vi "winchcontrol.vi"() -> ()   [LabVIEW 2009]
uses:
  Instance           1 20Saved   winchcontrol .vi
  Instance           2 20Saved   winchcontrol .vi
  Instance           4 20Saved   winchcontrol .vi
  Instance           3 20Saved   winchcontrol .vi
  Instance           5 20Saved   winchcontrol .vi
  Instance           6 20Saved   winchcontrol .vi
panel:
  out "Last update string":string
  in  "Port":i32=4050
  in  "Red Lion IP Address":string="192.168.1.160"
  in  "Beep\non wait?":bool=TRUE
  in  "Drive by \nCTD Data":bool
  out "isMaxPaySet":bool
  out "Old Max Payout":dbl
  in  "Maximum depth [m]":dbl=1000.0 min=0.0 max=2000.0 step=1.0 format="%#_4f"
  out "Time @ max":timestamp format="%<%H:%M:%S>T"
  out "Max payout":dbl format="%#_6f"
  out "Max depth":dbl format="%#_6f"
  in  "Go Up Now":bool
  in  "EMERGENCY\n      STOP":bool=TRUE caption="STOP!!!!!"
  in  "Final In Speed\n[turns/sec]":dbl=1.0 min=0.0 max=4.0 step=0.1 format="%_2f"
  in  "Slow depth\n[turns]":dbl=28.0 min=0.0 max=1500.0 step=1.0
  out "Final in Speed":dbl=3.0 min=0.0 max=4.0 step=0.1 format="%3_2g"
  out "Slow Depth":dbl=3.0 min=0.0 max=4.0 step=0.1
  out "Depth Derivative":dbl(graph)=-0.55843
  out "CTD Com Miss Count":dbl
  out "Winch Com Miss Count":dbl
  out "Sax Status":u8[](array[numeric])
  out "Pressure":dbl(graph)=-0.55843
  out "i value":i32
  out "concatenated string":string="$OPGST,1,2,1243"
  out "CTD data":string
  out "Depth":dbl(slide) min=0.0 max=1200.0 scale=2000.0..0.0 scale format="%#_4f"
  out "*(type *) &x":i32
  out "timestamp":u32=919485956
  out "Temperature":dbl(graph)=24.730053
  out "Parameter String":string="$OPGWPM,10,10,+0000,+0030,03,03,15000,15000,30000,30000,60000,60000,;"
  out "Status String":string="$OPGWST,1,0,2710.5,2710.5,0000, 00.00,-02,0000,ElmoStatusxxxxxx,;"
  out "Sax Status Code":dbl format="%#_8f"
  out "Motor Current":dbl=-2.0
  out "Motor Payout":dbl=2710.5
  out "Sheave Payout":dbl
  out "ATM90 Payout":dbl=2710.5
  in  "CTD Data  IP Address":string="192.168.1.158"
  in  "Port":i32=2342
  out "bytes written":i32
  out "RL Status Received":bool=TRUE
  out "Acc Out":dbl=15000.0
  out "Acc In":dbl=15000.0
  out "Winch Action Status":T1(ring)
  out "Winch Control Mode":T2(ring)=enum."MANUAL JOY"
  out "Decel Stop In":dbl=60000.0
  out "Decel Stop Out":dbl=60000.0
  out "Decel In":dbl=30000.0
  out "Decel Out":dbl=30000.0
  out "Wire In Speed":dbl=3.0
  out "Wire Out Speed":dbl=3.0
  out "Min Payout":dbl
  out "Max Payout":dbl=30.0
  out "I Limit Out":dbl=10.0
  out "I Limit In":dbl=10.0
  in  "Drop time [min.]":dbl=23.0 min=0.0 step=0.1 format="%.1f"
  out "output":string
  in  "Stop Now":bool
  in  "Wire In Speed\n[turns/sec]":dbl=2.8 min=0.0 max=5.0 step=0.1 format="%3_2f"
  in  "Decel in":dbl=30000.0
  in  "Decel out":dbl=30000.0
  in  "Stop decel in":dbl=60000.0
  in  "Stop decel out":dbl=60000.0
  in  "Accel  in":dbl=15000.0
  in  "Accel out":dbl=15000.0
  in  "Current limit out\n[Amps]":dbl=10.0 min=0.0 max=20.0 step=0.1 format="%_3f"
  in  "Current limit in\n[Amps]":dbl=16.0 min=0.0 max=18.0 format="%_3f"
  out "input 2":string="$OPGWPM,10,10,+0000,+0030,03,03,15000,15000,30000,30000,60000,60000,;"
  out "Depth History":cluster{"Depth":dbl, "Value":dbl}(graph)={"Depth"=0.0, "Value"=2710.5}
  out "Payout":dbl(slide)=97.75967413441958 min=0.0 max=1200.0 step=200.0 scale=2000.0..0.0 scale format="%#1_3f"
  out "Velocity Now":dbl(knob) min=-5.0 max=5.0 step=1.0 scale=-5.0..5.0 scale format="%#_1f"
  in  "Maximum payout [turns]":dbl=1500.0 min=0.0 max=1640.0 step=1.0 format="%#_4f"
  in  "Minimum payout [turns]":dbl=30.0 min=0.0 max=2000.0 step=1.0
  in  "Winch Auto Run":bool
  out "Enabled":bool
  in  "Wire Out Speed\n[turns/sec]":dbl=4.0 min=0.0 max=5.0 step=0.1 format="%_2f"
  out "Target\nDepth":dbl
  out "Conductivity":dbl(graph)=1e-06
  # "OPG  FAST  CTD"
  # "Winch Variable Status"
  # "Winch Variable Controls"
  # "FCTD DATA COMMUNICATION SETUP"
  # "RED LION CONTROL PANEL COM."
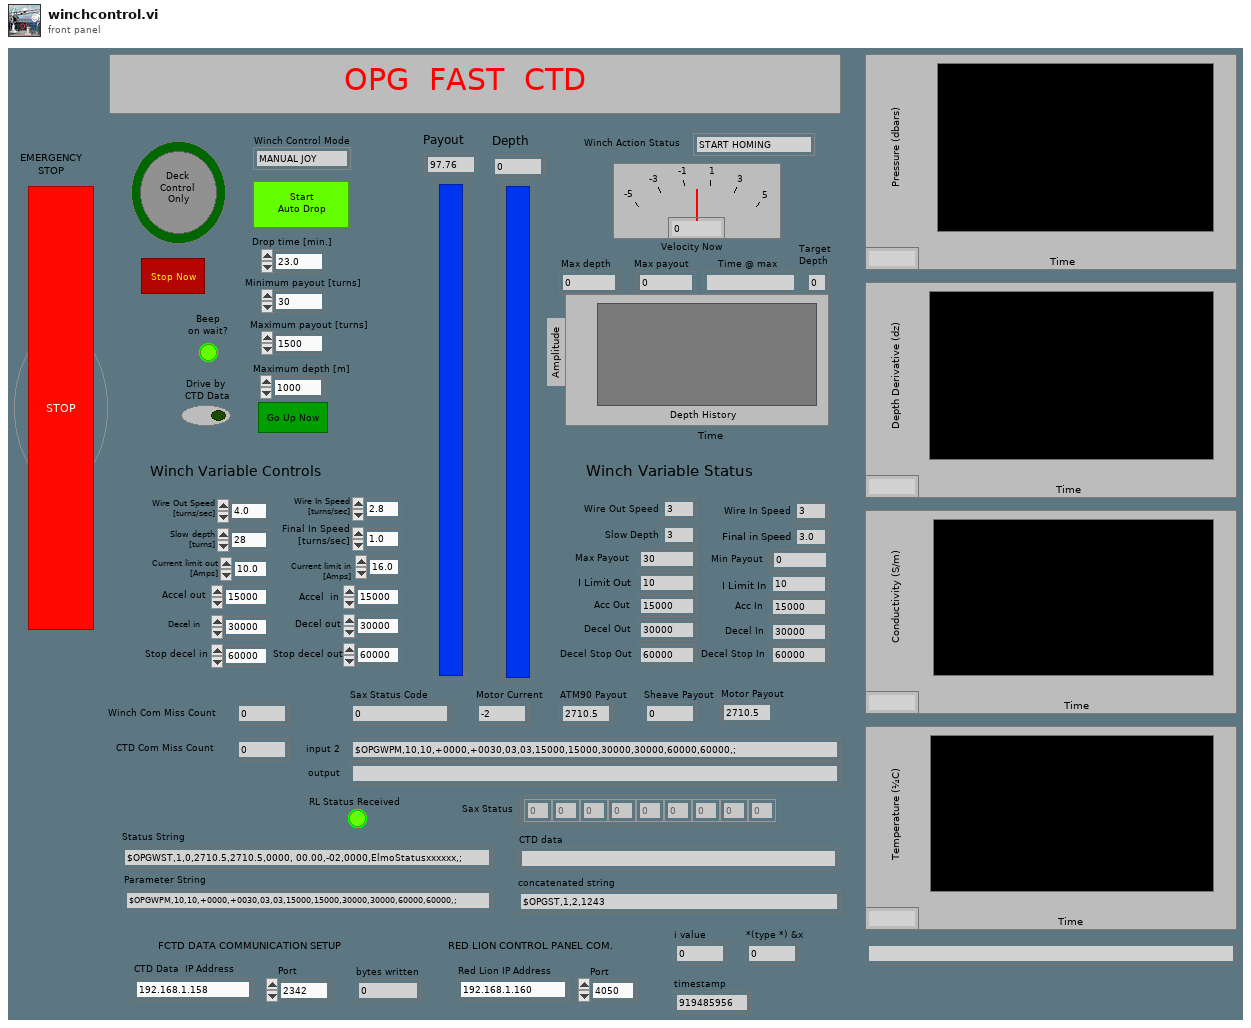
[diagram p1: front panel]
types:
  T1 = enum16{"START HOMING", "HOMING", "WAIT FOR TRIGGER", "START DROP", "GOING DOWN ?", "GOING UP"}
  T2 = enum16{"STOPPED", "MANUAL JOY", "MANUAL POT", "AUTO", "SEMIAUTO"}
  T3 = cluster{"Array[0]":dbl, "Array[1]":dbl, "Array[2]":dbl, "Array[3]":dbl, "Array[4]":dbl, "Array[5]":dbl, "Array[6]":dbl, "Array[7]":dbl, "Array[8]":dbl}
  T4 = cluster{"Array[0]":dbl, "Array[1]":dbl, "Array[2]":dbl, "Array[3]":dbl, "Array[4]":dbl, "Array[5]":dbl, "Array[6]":dbl, "Array[7]":dbl, "Array[8]":dbl, "Array[9]":dbl, "Array[10]":dbl, "Array[11]":dbl, "Array[12]":dbl, "Array[13]":dbl}
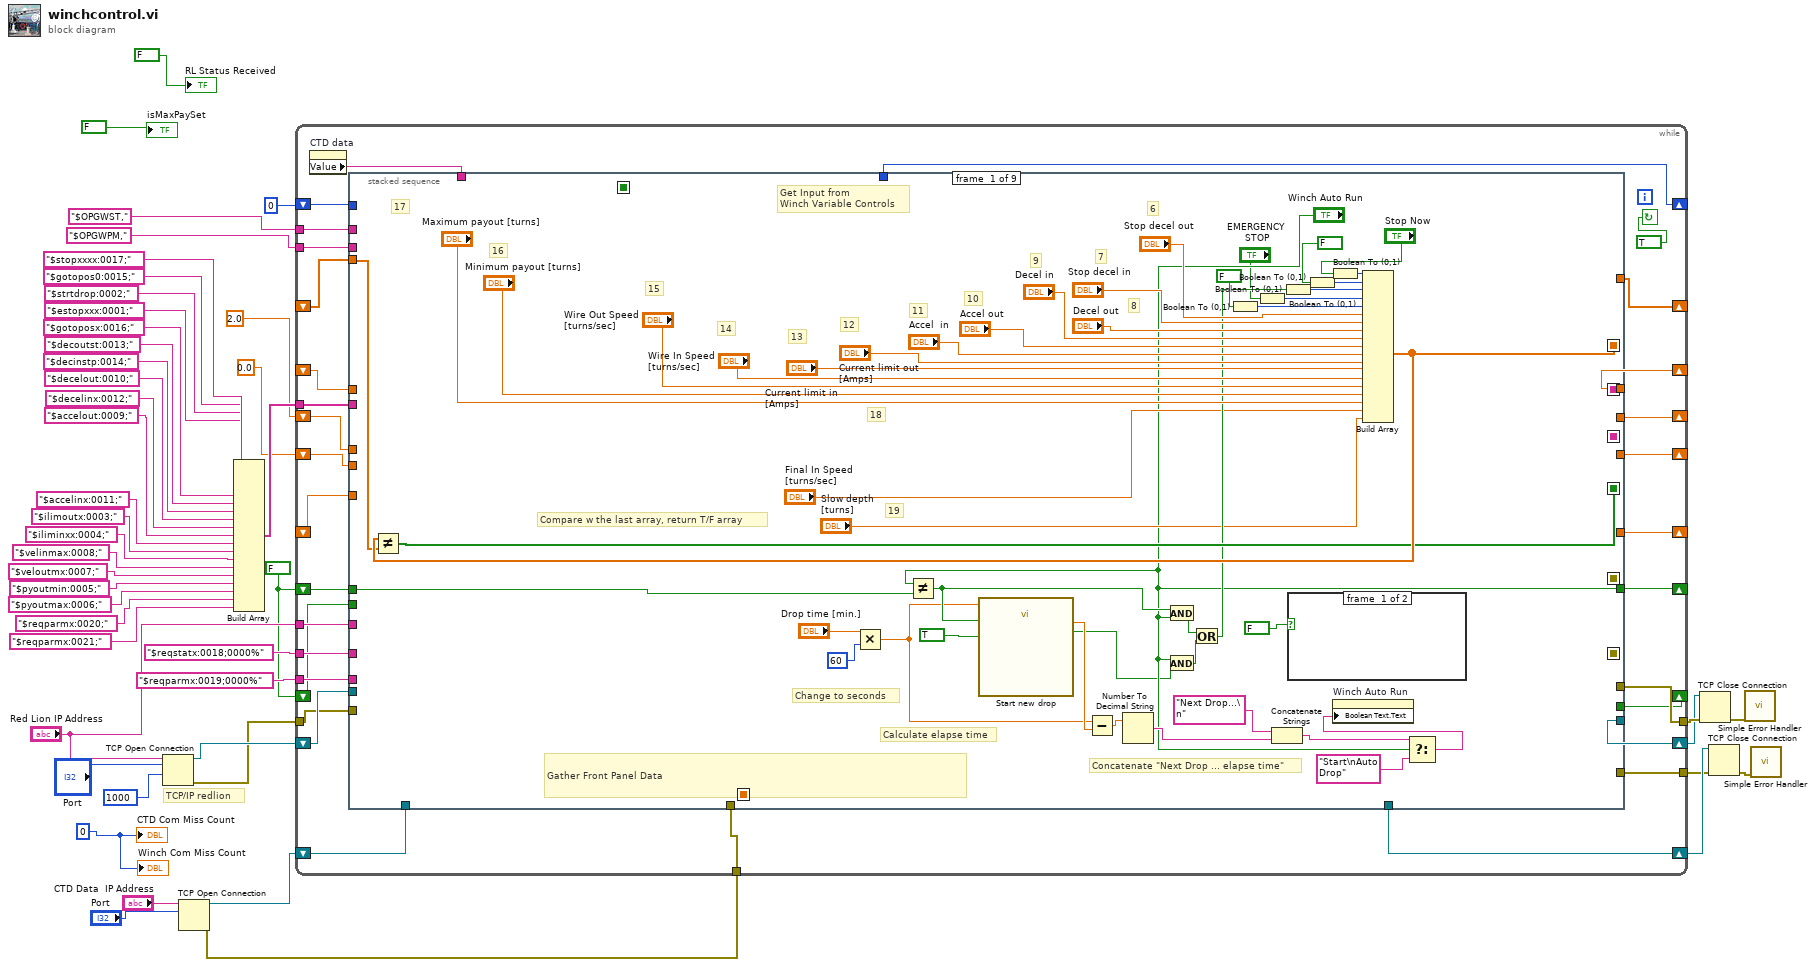
[diagram p0: block diagram]
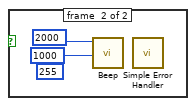
[diagram p2: hidden frame]
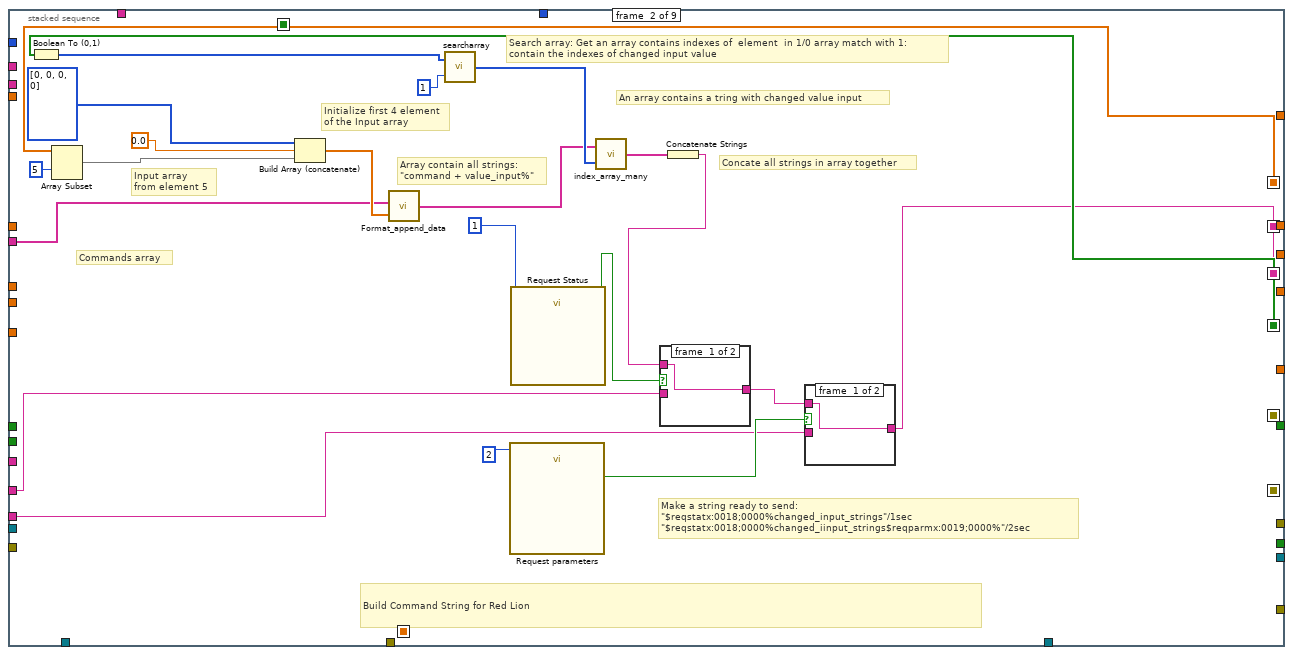
[diagram p3: hidden frame]
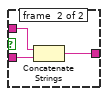
[diagram p4: hidden frame]
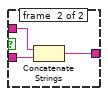
[diagram p5: hidden frame]
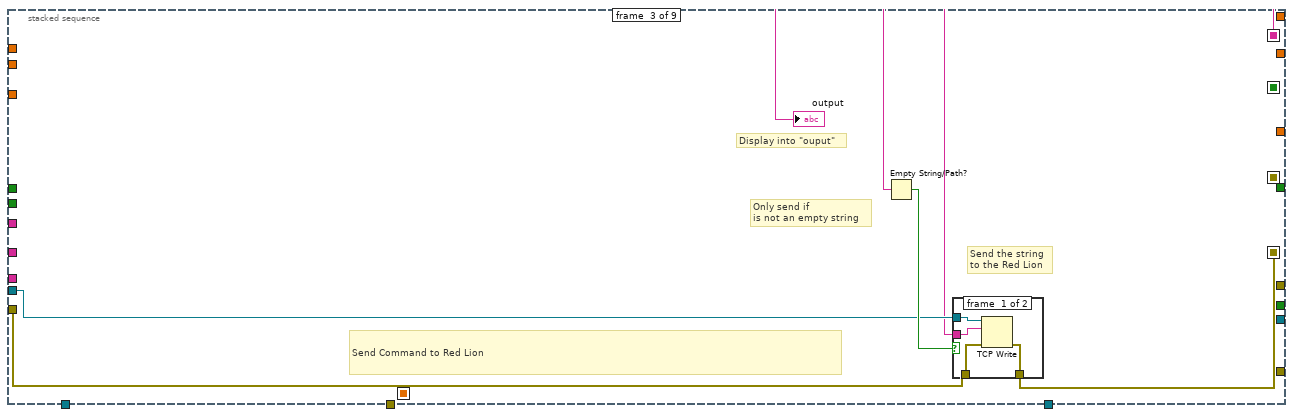
[diagram p6: hidden frame]
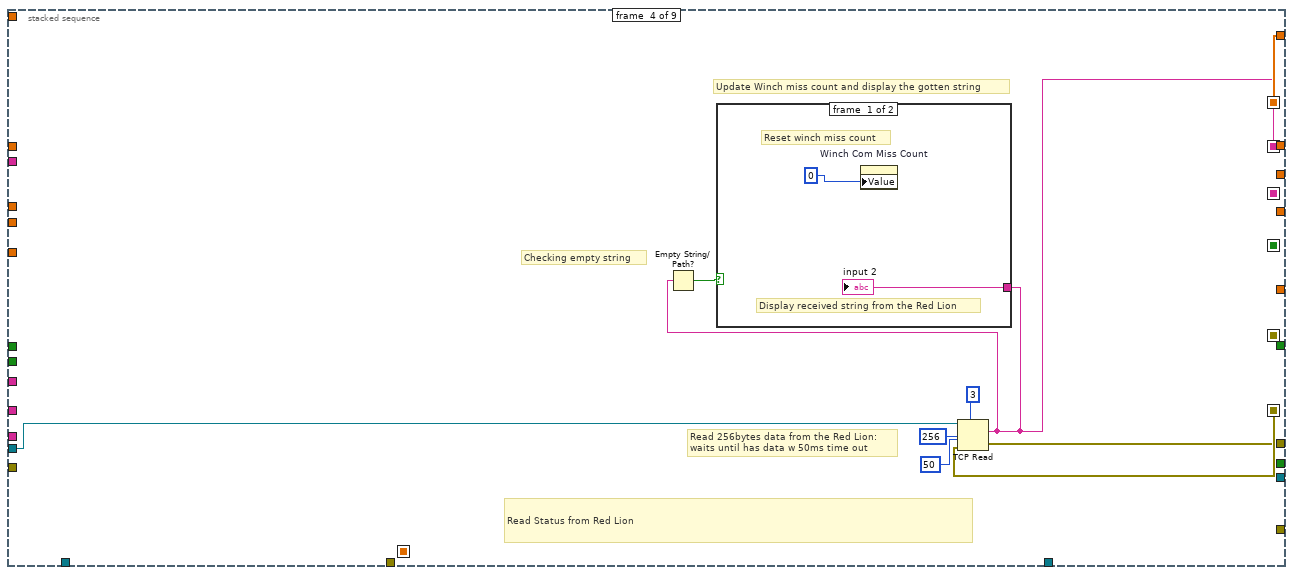
[diagram p8: hidden frame]
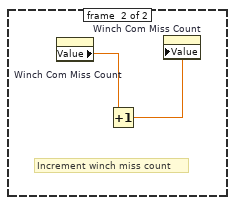
[diagram p9: hidden frame]
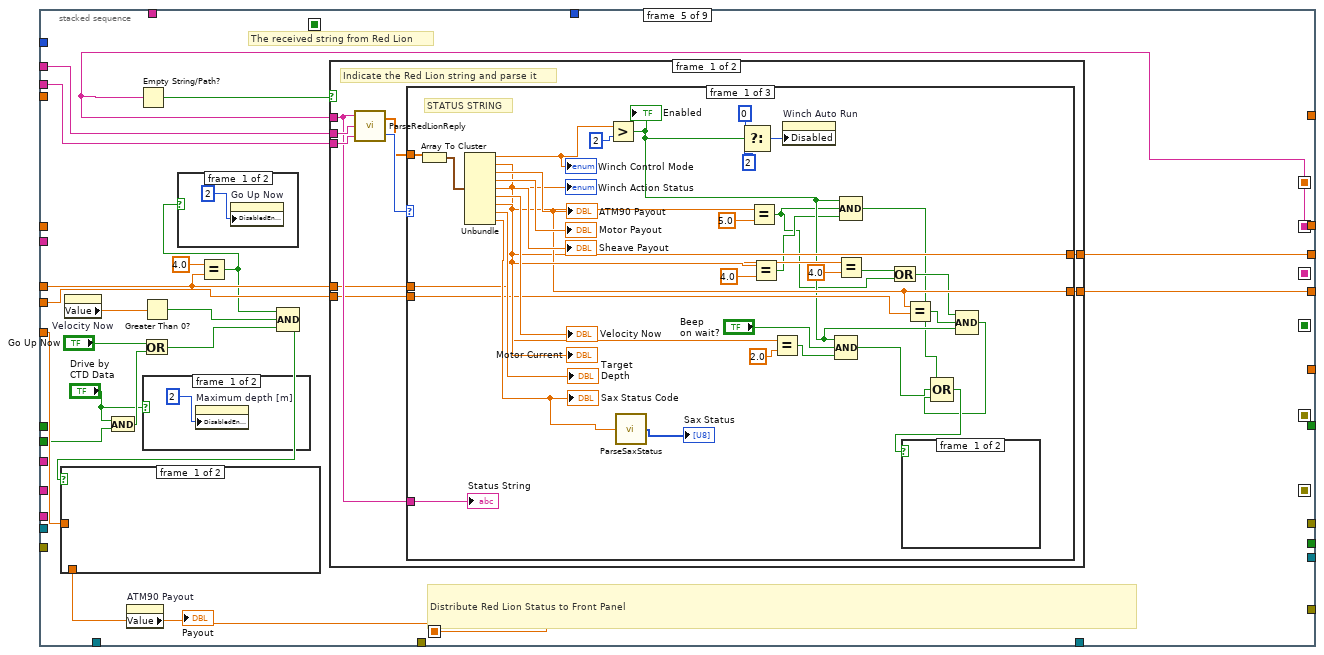
[diagram p10: hidden frame]
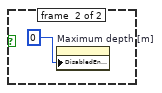
[diagram p11: hidden frame]
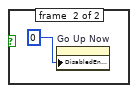
[diagram p12: hidden frame]
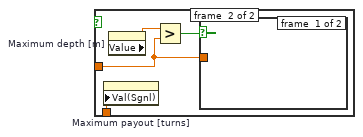
[diagram p13: hidden frame]
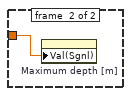
[diagram p14: hidden frame]
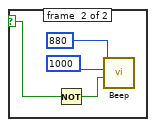
[diagram p15: hidden frame]
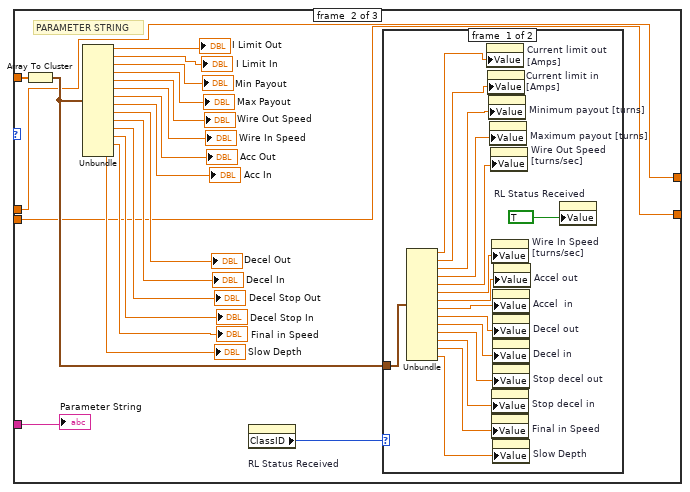
[diagram p16: hidden frame]
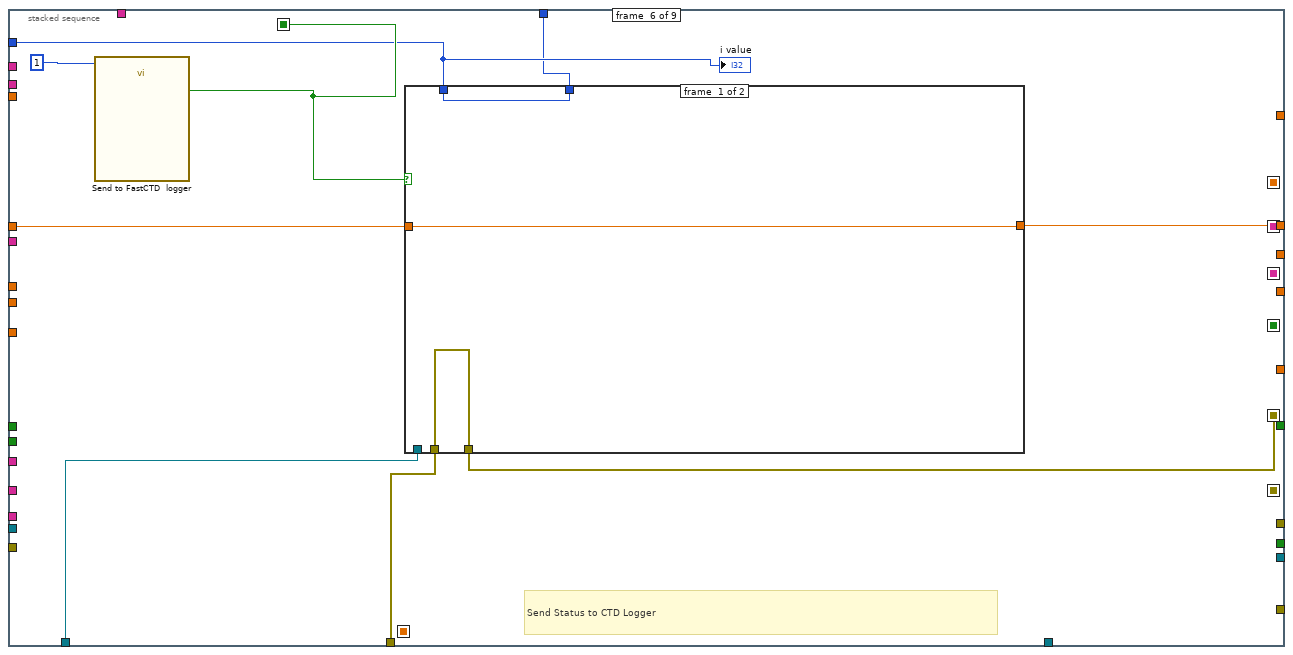
[diagram p20: hidden frame]
diagram:
  w3 = FALSE
  w10 = 0
  # "TCP/IP redlion"
  n1 = TCP Open Connection(address="Red Lion IP Address", remote port or service name="Port", timeout ms (60000)=1000) -> (connection ID=w45:refnum<k5>, error out=w43:errorcluster)  [unwired: 2 in]
  n2 = TCP Open Connection(address="CTD Data  IP Address", remote port or service name="Port") -> (connection ID=w19:refnum<k5>, error out=w17:errorcluster)  [unwired: 3 in]
  n3 = Build Array("$stopxxxx:0017;", "$gotopos0:0015;", "$strtdrop:0002;", "$estopxxx:0001;", "$gotoposx:0016;", "$decoutst:0013;", "$decinstp:0014;", "$decelout:0010;", "$decelinx:0012;", "$accelout:0009;", "$accelinx:0011;", "$ilimoutx:0003;", "$iliminxx:0004;", "$velinmax:0008;", "$veloutmx:0007;", "$pyoutmin:0005;", "$pyoutmax:0006;", "$reqparmx:0020;", "$reqparmx:0021;") -> (w41:string[])
  n4 = while {
    shift-right: [w78] -> _
    shift-left: _ -> [w76]
    tunnel: w43 -> [w73]
    tunnel: [w77] -> w42
    tunnel: w41 -> [w75]
    tunnel: "$reqstatx:0018;0000%" -> [w72]
    shift-right: [w71] -> _
    shift-left: w3 -> [w70]
    tunnel: w17 -> [w68]
    tunnel: [w67] -> w16
    tunnel: "$reqparmx:0019;0000%" -> [w66]
    shift-right: [w65] -> _
    shift-left: _ -> [w64]
    shift-right: [w63] -> _
    shift-left: 0 -> [w62]
    tunnel: "$OPGWST," -> [w61]
    tunnel: "$OPGWPM," -> [w60]
    shift-right: [w58] -> w9
    shift-left: w45 -> [w74]
    shift-right: [w57] -> w18
    shift-left: w19 -> [w69]
    shift-right: [w56] -> _
    shift-left: _ -> [w55]
    tunnel: "Red Lion IP Address" -> [w53]
    shift-right: [w52] -> _
    shift-left: w3 -> [w51]
    shift-right: [w50] -> _
    shift-left: 2.0 -> [w49]
    shift-right: [w48] -> _
    shift-left: 0.0 -> [w47]
    stop <- TRUE continue-if-true
    n5 = property on="CTD data" class="String"() -> ("Value"=w54:string)  [unwired: 2 in, 2 out]
    n6 = stacked-sequence {
      seq-local: [w123 _ _ _ _ _ _ _ _] -> [_ w140 _ w174 _ _ _ _ _]
      seq-local: [_ w126 _ _ _ _ _ _ _] -> [_ _ w156 _ _ _ _ _ _]
      seq-local: [_ _ w157 _ _ _ _ _ _] -> [_ _ _ w169 _ _ _ _ _]
      seq-local: [w119 _ _ _ _ _ _ _ _] -> [_ w147 _ _ _ _ _ _ _]
      seq-local: [_ _ _ w167 _ _ _ _ _] -> [_ _ _ _ w196 _ _ _ _]
      seq-local: [_ _ _ _ _ w302 _ _ _] -> [_ _ _ _ _ _ w348 _ _]
      seq-local: [_ _ _ _ w194 _ _ _ _] -> [_ _ _ _ _ _ w346 _ _]
      seq-local: [_ _ _ _ _ w301 _ _ _] -> [_ _ _ _ _ _ w345 _ _]
      tunnel: w73 -> [_ _ w159 _ _ _ _ _ _]
      tunnel: w74 -> [_ _ w158 w170 _ _ _ w436 _]
      tunnel: [_ _ _ w174 _ _ _ _ _] -> w78
      tunnel: w75 -> [_ w138 _ _ _ _ _ _ _]
      tunnel: [_ _ _ w168 _ _ _ _ _] -> w77
      tunnel: w76 -> [w122 _ _ _ _ _ _ _ _]
      tunnel: w72 -> [_ w132 _ _ _ _ _ _ _]
      tunnel: ["Winch Auto Run" _ _ _ _ _ _ _ _] -> w71
      tunnel: w70 -> [w97 _ _ _ _ _ _ _ _]
      tunnel: w69 -> [_ _ _ _ _ w304 w349 w434 _]
      tunnel: w68 -> [_ _ _ _ _ w303 _ _ _]
      tunnel: [_ _ _ _ _ _ w347 _ _] -> w67
      tunnel: w66 -> [_ w127 _ _ _ _ _ _ _]
      tunnel: [_ _ _ _ _ w299 _ _ _] -> w65
      tunnel: w64 -> [_ _ _ _ _ w298 _ _ _]
      tunnel: w62 -> [_ _ _ _ _ w297 _ _ _]
      tunnel: [_ _ _ _ _ w296 _ _ _] -> w63
      tunnel: w61 -> [_ _ _ _ w198 _ _ _ _]
      tunnel: w60 -> [_ _ _ _ w197 _ _ _ _]
      tunnel: [_ _ _ _ _ _ _ w435 _] -> w58
      tunnel: [_ _ _ _ _ _ _ w433 _] -> w57
      tunnel: [_ _ _ _ _ _ w344 _ _] -> w56
      tunnel: w55 -> [_ _ _ _ w190 _ w343 _ _]
      tunnel: w54 -> [_ _ _ _ _ _ w342 _ _]
      tunnel: w53 -> [_ _ _ _ _ _ _ w432 _]
      tunnel: [_ _ _ _ _ _ w341 _ _] -> w52
      tunnel: w51 -> [_ _ _ _ w187 _ _ _ _]
      tunnel: [_ _ _ _ w184 _ _ _ _] -> w50
      tunnel: w49 -> [_ _ _ _ w180 _ _ _ _]
      tunnel: [_ _ _ _ w183 _ _ _ _] -> w48
      tunnel: w47 -> [_ _ _ _ w182 _ _ _ _]
      frame #0 {
        w120 = FALSE items=["OFF", "ON", "OFF", "ON"] ("Return to top")
        w106 = FALSE items=["OFF", "ON", "OFF", "ON"] ("Go to ...")
        # "19"
        # "18"
        # "17"
        # "16"
        # "15"
        # "14"
        # "13"
        # "12"
        # "11"
        # "10"
        # "9"
        # "8"
        # "7"
        # "6"
        # "Compare w the last array, return T/F array"
        # "Concatenate \"Next Drop ... elapse time\""
        # "Calculate elapse time"
        # "Change to seconds"
        # "Get Input from\nWinch Variable Controls"
        # "Gather Front Panel Data"
        n7 = Multiply(x="Drop time [min.]", y=60) -> (x*y=w91:dbl)
        n8 = Not Equal?(x="Winch Auto Run", y=w97) -> (x != y?=w96:bool)
        n9 = call "Start new drop"("Time Target (s)"=w91, "Reset"=w96, "Auto Reset"=TRUE) -> ("Elapsed Time (s)"=w92:dbl, "Time has Elapsed"=w81:bool)  [unwired: 9 in, 6 out]
        n10 = Subtract(x=w91, y=w92) -> (x-y=w90:dbl)
        n11 = Number To Decimal String(number=w90) -> (decimal integer string=w89:string)  [unwired: 1 in]
        n12 = And(x=w96, y="Winch Auto Run") -> (x .and. y?=w95:bool)
        n13 = And(x="Winch Auto Run", y=w81) -> (x .and. y?=w94:bool)
        n14 = Or(x=w95, y=w94) -> (x .or. y?=w93:bool)
        n15 = Boolean To (0,1)(Boolean=w106) -> (0, 1=w105:i16)
        n16 = Boolean To (0,1)(Boolean="EMERGENCY\n      STOP") -> (0, 1=w104:i16)
        n17 = Concatenate Strings("Next Drop...\n", w89) -> (w86:string)
        n18 = Boolean To (0,1)(Boolean=w93) -> (0, 1=w103:i16)
        n19 = case shown="True" FALSE {
          frame #0 {
          }
          frame #1 {
            (unwired) 255
            n20 = call <vilib>:"Beep.vi"("duration (msec) - ignored"=1000, "frequency (Hz) - ignored"=2000) -> ()  [unwired: 10 in]
            n21 = call <vilib>:"Simple Error Handler.vi"() -> ()  [unwired: 5 in, 5 out]
          }
        }
        n22 = Boolean To (0,1)(Boolean=w120) -> (0, 1=w102:i16)
        n23 = Boolean To (0,1)(Boolean="Stop Now") -> (0, 1=w101:i16)
        n24 = Build Array(w101, w102, w103, w104, w105, "Stop decel out", "Stop decel in", "Decel out", "Decel in", "Accel out", "Accel  in", "Current limit out\n[Amps]", "Current limit in\n[Amps]", "Wire In Speed\n[turns/sec]", "Wire Out Speed\n[turns/sec]", "Minimum payout [turns]", "Maximum payout [turns]", "Final In Speed\n[turns/sec]", "Slow depth\n[turns]") -> (w123:dbl[])
        n25 = Not Equal?(x=w123, y=w122) -> (x != y?=w119:bool[])
        n26 = Select(t=w86, s="Winch Auto Run", f="Start\nAuto Drop") -> (s? t:f=w87:string)
        n27 = property on="Winch Auto Run" class="Bool (strict)"("Boolean Text.Text"=w87) -> ()  [unwired: 2 in, 2 out]
      }
      frame #1 {
        # "Make a string ready to send:\n\"$reqstatx:0018;0000%changed_input_strings\"/1sec\n\"$reqstatx:0018;0000%changed_iinput_strings$reqparmx:0019;0000%\"/2sec"
        # "Concate all strings in array together"
        # "An array contains a tring with changed value input"
        # "Array contain all strings:\n\"command + value_input%\""
        # "Commands array"
        # "Initialize first 4 element\nof the Input array"
        # "Input array\nfrom element 5"
        # "Search array: Get an array contains indexes of  element  in 1/0 array match with 1:\ncontain the indexes of changed input value"
        # "Build Command String for Red Lion"
        n28 = Boolean To (0,1)(Boolean=w147) -> (0, 1=w145:i16[])
        n29 = Array Subset(array=w140, index=5) -> (w136:dbl[])  [unwired: 1 in]
        n30 = Build Array (concatenate)(i32[] [0, 0, 0, 0], 0.0 ("Depth to go to"), w136) -> (w139:dbl[])
        n31 = call "Format_append_data.vi"("Numbers to append"=w139, "Strings without numbers"=w138) -> ("Final Strings"=w137:string[])
        n32 = call "searcharray.vi"("Search character"=1, "Array 2"=w145) -> ("Array"=w144:i16[])
        n33 = call "Request parameters"("Time Target (s)"=2) -> ("Time has Elapsed"=w128:bool)  [unwired: 11 in, 7 out]
        n34 = call "Request Status"("Time Target (s)"=1) -> ("Time has Elapsed"=w133:bool)  [unwired: 11 in, 7 out]
        n35 = call "index_array_many.vi"("Lines of Array to grab"=w144, "String Array Input"=w137) -> ("Output array"=w143:string[])
        n36 = Concatenate Strings(w143) -> (w131:string)
        n37 = case shown="True" w133 {
          tunnel: w131 -> [w152 w155]
          tunnel: [w152 w154] -> w129
          tunnel: w132 -> [_ w153]
          frame #0 {
          }
          frame #1 {
            n38 = Concatenate Strings(w155, w153) -> (w154:string)
          }
        }
        n39 = case shown="True" w128 {
          tunnel: w129 -> [w148 w151]
          tunnel: [w148 w150] -> w126
          tunnel: w127 -> [_ w149]
          frame #0 {
          }
          frame #1 {
            n40 = Concatenate Strings(w151, w149) -> (w150:string)
          }
        }
      }
      frame #2 {
        # "Send the string\nto the Red Lion"
        # "Only send if\nis not an empty string"
        # "Display into \"ouput\""
        # "Send Command to Red Lion"
        n41 = Empty String/Path?(string/path=w156) -> (empty?=w160:bool)
        n42 = case shown="False" w160 {
          tunnel: w156 -> [w163 _]
          tunnel: w158 -> [w164 _]
          tunnel: w159 -> [w162 w165]
          tunnel: [w161 w165] -> w157
          frame #0 {
            n43 = TCP Write(connection ID=w164, data in=w163, error in (no error)=w162) -> (error out=w161:errorcluster)  [unwired: 1 in, 2 out]
          }
          frame #1 {
          }
        }
        "output" <- w156
      }
      frame #3 {
        # "Update Winch miss count and display the gotten string"
        # "Checking empty string"
        # "Read 256bytes data from the Red Lion:\nwaits until has data w 50ms time out"
        # "Read Status from Red Lion"
        n44 = TCP Read(connection ID=w170, bytes to read=256, error in (no error)=w169, 7:3, 9:50) -> (data out=w167:string, error out=w168:errorcluster)  [unwired: 1 out]
        n45 = Empty String/Path?(string/path=w167) -> (empty?=w166:bool)
        n46 = case shown="False" w166 {
          tunnel: w167 -> [w176 _]
          frame #0 {
            # "Display received string from the Red Lion"
            # "Reset winch miss count"
            n47 = property on="Winch Com Miss Count" class="DigNum (strict)"("Value"=0) -> ()  [unwired: 2 in, 2 out]
            "input 2" <- w176
          }
          frame #1 {
            # "Increment winch miss count"
            n48 = property on="Winch Com Miss Count" class="DigNum (strict)"() -> ("Value"=w178:dbl)  [unwired: 2 in, 2 out]
            n49 = Increment(x=w178) -> (x+1=w177:dbl)
            n50 = property on="Winch Com Miss Count" class="DigNum (strict)"("Value"=w177) -> ()  [unwired: 2 in, 2 out]
          }
        }
      }
      frame #4 {
        # "The received string from Red Lion"
        # "Distribute Red Lion Status to Front Panel"
        n51 = property on="Velocity Now" class="Knob (strict)"() -> ("Value"=w193:dbl)  [unwired: 2 in, 2 out]
        n52 = And(x="Drive by \nCTD Data", y=w187) -> (x .and. y?=w186:bool)
        n53 = property on="ATM90 Payout" class="Digital (strict)"() -> ("Value"=w194:dbl)  [unwired: 2 in, 2 out]
        "Payout" <- w194
        n54 = Empty String/Path?(string/path=w196) -> (empty?=w195:bool)
        n55 = Greater Than 0?(x=w193) -> (x > 0?=w191:bool)
        n56 = Or(x="Go Up Now", y=w186) -> (x .or. y?=w188:bool)
        n57 = case shown="False" "Drive by \nCTD Data" {
          frame #0 {
            n58 = property on="Maximum depth [m]" class="DigNum (strict)"("DisabledEnum"=2) -> ()  [unwired: 2 in, 2 out]
          }
          frame #1 {
            n59 = property on="Maximum depth [m]" class="DigNum (strict)"("DisabledEnum"=0) -> ()  [unwired: 2 in, 2 out]
          }
        }
        n60 = Equal?(x=4.0, y=w180) -> (x = y?=w179:bool)
        n61 = case shown="True" w179 {
          frame #0 {
            n62 = property on="Go Up Now" class="Bool"("DisabledEnum"=2) -> ()  [unwired: 2 in, 2 out]
          }
          frame #1 {
            n63 = property on="Go Up Now" class="Bool"("DisabledEnum"=0) -> ()  [unwired: 2 in, 2 out]
          }
        }
        n64 = Compound Arithmetic op=AND(w179, w191, w188) -> (w192:bool)
        n65 = case shown="True" w192 {
          tunnel: w194 -> [_ w206]
          tunnel: w190 -> [_ w203]
          frame #0 {
          }
          frame #1 {
            n66 = property on="Maximum payout [turns]" class="DigNum (strict)"("Val(Sgnl)"=w206) -> ()  [unwired: 2 in, 2 out]
            n67 = property on="Maximum depth [m]" class="DigNum (strict)"() -> ("Value"=w205:dbl)  [unwired: 2 in, 2 out]
            n68 = Greater?(x=w205, y=w203) -> (0:w204:bool)
            n69 = case shown="True" w204 {
              tunnel: w203 -> [_ w207]
              frame #0 {
              }
              frame #1 {
                n70 = property on="Maximum depth [m]" class="DigNum (strict)"("Val(Sgnl)"=w207) -> ()  [unwired: 2 in, 2 out]
              }
            }
          }
        }
        n71 = case shown="False" w195 {
          tunnel: w198 -> [w214 _]
          tunnel: w197 -> [w213 _]
          tunnel: w196 -> [w212 _]
          tunnel: [w211 w295] -> w184
          tunnel: w180 -> [w210 w295]
          tunnel: [w209 w294] -> w183
          tunnel: w182 -> [w208 w294]
          frame #0 {
            # "Indicate the Red Lion string and parse it"
            n72 = call "ParseRedLionReply.vi"("Parameter Iidicator"=w213, "Status Indicator"=w214, "Red Lion String"=w212) -> ("Type"=w216:i16, "Array"=w215:dbl[])
            n73 = case shown="0" w216 {
              tunnel: w215 -> [w250 w275 _]
              tunnel: w212 -> [w242 w261 _]
              tunnel: [w229 w258 w293] -> w211
              tunnel: w210 -> [w233 w258 w293]
              tunnel: [w232 w257 w292] -> w209
              tunnel: w208 -> [w231 w257 w292]
              frame #0 {
                # "STATUS STRING"
                n74 = Array To Cluster(array=w250) -> (cluster=w249:T3)
                n75 = Unbundle(w249) -> ("Array[0]"=w248:dbl, "Array[1]"=w229:dbl, "Array[2]"=w232:dbl, "Array[3]"=→"Motor Payout":dbl, "Array[4]"=→"Sheave Payout":dbl, "Array[5]"=→"Velocity Now":dbl, "Array[6]"=→"Motor Current":dbl, "Array[7]"=→"Target\nDepth":dbl, "Array[8]"=w238:dbl)
                "Winch Control Mode" <- w248
                "Winch Action Status" <- w229
                "ATM90 Payout" <- w232
                "Sax Status Code" <- w238
                n76 = Greater?(x=w248, y=2) -> (0:w225:bool)
                "Enabled" <- w225
                n77 = call "ParseSaxStatus.vi"("Status Code In"=w238) -> ("Status Flags"=→"Sax Status":i8[])
                n78 = Select(t=0, s=w225, f=2) -> (s? t:f=w239:i32)
                n79 = Equal?(x=w229, y=5.0) -> (x = y?=w218:bool)
                n80 = Equal?(x=w233, y=4.0) -> (x = y?=w222:bool)
                n81 = Equal?(x=w229, y=2.0) -> (x = y?=w224:bool)
                n82 = property on="Winch Auto Run" class="Boolean (strict)"("Disabled"=w239) -> ()  [unwired: 2 in, 2 out]
                n83 = Compound Arithmetic op=AND(w225, "Beep\non wait?", w224) -> (w219:bool)
                n84 = Equal?(x=w229, y=4.0) -> (x = y?=w228:bool)
                n85 = Compound Arithmetic op=AND(w225, w218, w222) -> (w221:bool)
                n86 = Or(x=w228, y=w218) -> (x .or. y?=w227:bool)
                n87 = Equal?(x=w232, y=w231) -> (x = y?=w226:bool)
                n88 = Compound Arithmetic op=AND(w227, w226, w225) -> (w217:bool)
                n89 = Compound Arithmetic op=OR(w221, w219, w217) -> (w220:bool)
                n90 = case shown="True" w220 {
                  selector: w220 -> [_ w252]
                  frame #0 {
                  }
                  frame #1 {
                    n91 = Not(x=w252) -> (.not. x?=w253:bool)
                    n92 = call <vilib>:"Beep.vi"("use system alert? (T) - ignored"=w253, "duration (msec) - ignored"=u32 1000, "frequency (Hz) - ignored"=u32 880) -> ()  [unwired: 9 in]
                  }
                }
                "Status String" <- w242
              }
              frame #1 {
                # "PARAMETER STRING"
                n93 = Array To Cluster(array=w275) -> (cluster=w262:T4)
                n94 = Unbundle(w262) -> ("Array[0]"=→"I Limit Out":dbl, "Array[1]"=→"I Limit In":dbl, "Array[2]"=→"Min Payout":dbl, "Array[3]"=→"Max Payout":dbl, "Array[4]"=→"Wire Out Speed":dbl, "Array[5]"=→"Wire In Speed":dbl, "Array[6]"=→"Acc Out":dbl, "Array[7]"=→"Acc In":dbl, "Array[8]"=→"Decel Out":dbl, "Array[9]"=→"Decel In":dbl, "Array[10]"=→"Decel Stop Out":dbl, "Array[11]"=→"Decel Stop In":dbl, "Array[12]"=→"Final in Speed":dbl, "Array[13]"=→"Slow Depth":dbl)
                n95 = property on="RL Status Received" class="Bool (strict)"() -> ("ClassID"=w256:u32)  [unwired: 2 in, 2 out]
                n96 = case shown="0, Default" w256 {
                  tunnel: w262 -> [w291 _]
                  frame #0 {
                    n97 = Unbundle(w291) -> ("Array[0]"=w290:dbl, "Array[1]"=w289:dbl, "Array[2]"=w288:dbl, "Array[3]"=w287:dbl, "Array[4]"=w286:dbl, "Array[5]"=w285:dbl, "Array[6]"=w279:dbl, "Array[7]"=w284:dbl, "Array[8]"=w283:dbl, "Array[9]"=w282:dbl, "Array[10]"=w281:dbl, "Array[11]"=w280:dbl, "Array[12]"=w278:dbl, "Array[13]"=w277:dbl)
                    n98 = property on="Current limit out\n[Amps]" class="DigNum (strict)"("Value"=w290) -> ()  [unwired: 2 in, 2 out]
                    n99 = property on="Current limit in\n[Amps]" class="DigNum (strict)"("Value"=w289) -> ()  [unwired: 2 in, 2 out]
                    n100 = property on="Minimum payout [turns]" class="DigNum (strict)"("Value"=w288) -> ()  [unwired: 2 in, 2 out]
                    n101 = property on="Maximum payout [turns]" class="DigNum (strict)"("Value"=w287) -> ()  [unwired: 2 in, 2 out]
                    n102 = property on="Wire Out Speed\n[turns/sec]" class="DigNum (strict)"("Value"=w286) -> ()  [unwired: 2 in, 2 out]
                    n103 = property on="Wire In Speed\n[turns/sec]" class="DigNum (strict)"("Value"=w285) -> ()  [unwired: 2 in, 2 out]
                    n104 = property on="Stop decel in" class="DigNum (strict)"("Value"=w280) -> ()  [unwired: 2 in, 2 out]
                    n105 = property on="Final in Speed" class="DigNum (strict)"("Value"=w278) -> ()  [unwired: 2 in, 2 out]
                    n106 = property on="Accel  in" class="DigNum (strict)"("Value"=w284) -> ()  [unwired: 2 in, 2 out]
                    n107 = property on="Decel out" class="DigNum (strict)"("Value"=w283) -> ()  [unwired: 2 in, 2 out]
                    n108 = property on="Decel in" class="DigNum (strict)"("Value"=w282) -> ()  [unwired: 2 in, 2 out]
                    n109 = property on="Stop decel out" class="DigNum (strict)"("Value"=w281) -> ()  [unwired: 2 in, 2 out]
                    n110 = property on="Slow Depth" class="DigNum (strict)"("Value"=w277) -> ()  [unwired: 2 in, 2 out]
                    n111 = property on="Accel out" class="DigNum (strict)"("Value"=w279) -> ()  [unwired: 2 in, 2 out]
                    n112 = property on="RL Status Received" class="Bool (strict)"("Value"=TRUE) -> ()  [unwired: 2 in, 2 out]
                  }
                  frame #1 {
                  }
                }
                "Parameter String" <- w261
              }
              frame #2 {
                # "INVALID STRING"
              }
            }
          }
          frame #1 {
            # "If empty string, do nothing"
          }
        }
      }
      frame #5 {
        # "Send Status to CTD Logger"
        n113 = call "Send to FastCTD  logger"("Time Target (s)"=1) -> ("Time has Elapsed"=w301:bool)  [unwired: 11 in, 7 out]
        n114 = case shown="True" w301 {
          tunnel: w304 -> [_ w317]
          tunnel: w303 -> [w307 w316]
          tunnel: [w307 w315] -> w302
          tunnel: [w306 w311] -> w299
          tunnel: w298 -> [w306 w310]
          tunnel: w297 -> [w305 w309]
          tunnel: [w305 w308] -> w296
          frame #0 {
          }
          frame #1 {
            n115 = property on="Status String" class="String"() -> ("Value"=w313:string)  [unwired: 2 in, 2 out]
            n116 = Empty String/Path?(string/path=w313) -> (empty?=w314:bool)
            n117 = case shown="True" w314 {
              tunnel: w313 -> [w321 _]
              tunnel: [w321 w331] -> w312
              tunnel: [w320 w325] -> w311
              tunnel: w310 -> [w320 w324]
              tunnel: w309 -> [w319 w323]
              tunnel: [w319 w322] -> w308
              frame #0 {
              }
              frame #1 {
                # "Since Status string is empty, make a string \"$OPGST,1,2/3,1243\"\nto send to FCTD app"
                n118 = Increment(x=w323) -> (x+1=w322:i32)
                n119 = Quotient & Remainder(x=w322, y=4) -> (x-y*floor(x/y)=w328:i32)  [unwired: 1 out]
                n120 = Equal To 0?(x=w328) -> (x = 0?=w327:bool)
                n121 = case shown="False" w327 {
                  tunnel: [w334 w336] -> w326
                  tunnel: [w334 w336] -> w325
                  tunnel: w324 -> [w334 w335]
                  frame #0 {
                  }
                  frame #1 {
                    n122 = Equal?(x=w335, y=3.0) -> (x = y?=w337:bool)
                    n123 = Select(t=2.0 ("y"), s=w337, f=3.0 ("y")) -> (s? t:f=w336:dbl)
                  }
                }
                n124 = Number To Decimal String(number=w326) -> (decimal integer string=w330:string)  [unwired: 1 in]
                n125 = Concatenate Strings("$OPGST,1," ("string"), w330, ",1243" ("string")) -> (w331:string)
                "concatenated string" <- w331
              }
            }
            n126 = TCP Write(connection ID=w317, data in=w312, error in (no error)=w316) -> (bytes written=→"bytes written":i32, error out=w315:errorcluster)  [unwired: 1 in, 1 out]
          }
        }
        "i value" <- w297
      }
      frame #6 {
        # "Every one second"
        # "Read Data from CTD Logger"
        n127 = case shown="True" w345 {
          selector: w345 -> [w350 _]
          tunnel: w349 -> [_ w373]
          tunnel: w348 -> [w352 w354]
          tunnel: [w352 w362] -> w347
          tunnel: w346 -> [_ w372]
          tunnel: [w351 w358] -> w344
          tunnel: w343 -> [w351 w357]
          tunnel: w342 -> [_ w355]
          tunnel: [w350 w353] -> w341
          frame #0 {
          }
          frame #1 {
            w371 = 4
            # "Read CTD\ndata"
            # "Receive\nCTD length"
            n128 = TCP Read(connection ID=w373, bytes to read=w371, error in (no error)=w354) -> (connection ID out=w370:refnum<k5>, data out=w369:string, error out=w367:errorcluster)  [unwired: 2 in]
            n129 = Type Cast(type=w371, x=w369) -> (*(type *) &x=w368:i32)
            "*(type *) &x" <- w368
            n130 = TCP Read(connection ID=w370, bytes to read=w368, error in (no error)=w367) -> (connection ID out=w361:refnum<k5>, data out=w356:string, error out=w363:errorcluster)  [unwired: 2 in]
            "CTD data" <- w356
            n131 = Equal?(x=w355, y=w356) -> (x = y?=w353:bool)
            n132 = property on="Pressure" class="WFChart (strict)"("Blinking"=w353) -> ()  [unwired: 2 in, 2 out]
            n133 = property on="Depth Derivative" class="WFChart (strict)"("Blinking"=w353) -> ()  [unwired: 2 in, 2 out]
            n134 = property on="Conductivity" class="WFChart (strict)"("Blinking"=w353) -> ()  [unwired: 2 in, 2 out]
            n135 = property on="Temperature" class="WFChart (strict)"("Blinking"=w353) -> ()  [unwired: 2 in, 2 out]
            n136 = property on="Depth" class="Slide (strict)"("Blinking"=w353) -> ()  [unwired: 2 in, 2 out]
            n137 = property on="CTD data" class="Str"("Blinking"=w353) -> ()  [unwired: 2 in, 2 out]
            n138 = Empty String/Path?(string/path=w356) -> (empty?=w365:bool)
            n139 = TCP Read(connection ID=w361, error in (no error)=w363, 7:3, 9:5) -> (error out=w362:errorcluster)  [unwired: 1 in, 2 out]
            n140 = case shown="False" w365 {
              tunnel: w356 -> [w387 _]
              tunnel: [w374 0.0] -> w366
              tunnel: [w374 w429] -> w358
              tunnel: w357 -> [w388 w429]
              frame #0 {
                # "Otherwise, has CTD data, parse it and display temp, pressure, conductivity"
                n141 = property on="CTD Com Miss Count" class="DigNum (strict)"("Value"=0) -> ()  [unwired: 2 in, 2 out]
                n142 = property on="Winch Action Status" class="Enum (strict)"() -> ("Value"=w381:T1)  [unwired: 2 in, 2 out]
                n143 = Scan From String(format string="%d,%f,%f,%f", input string=w387, initial scan location=u32 0) -> (output 1=→"timestamp":u32, output 2=w382:dbl, output 3=→"Temperature":dbl, output 4=→"Conductivity":dbl)  [unwired: 5 in, 3 out]
                "Pressure" <- w382
                n144 = Greater?(x=w381, y=3) -> (0:w376:bool)
                n145 = call "Press2Depth.vi"("Pressure in dbars"=w382) -> ("Depth in meters"=w374:dbl)
                "Depth" <- w374
                n146 = Subtract(x=w388, y=w374) -> (x-y=→"Depth Derivative":dbl)
                n147 = property on="Drive by \nCTD Data" class="Bool (strict)"() -> ("Value"=w383:bool)  [unwired: 2 in, 2 out]
                n148 = property on="Max depth" class="DigNum (strict)"() -> ("Value"=w379:dbl)  [unwired: 2 in, 2 out]
                n149 = Greater?(x=w374, y="Maximum depth [m]") -> (0:w384:bool)
                n150 = And(x=w384, y=w383) -> (x .and. y?=w385:bool)
                n151 = stacked-sequence {
                  tunnel: [w396 _] -> _
                  tunnel: w374 -> [_ w414]
                  tunnel: "Maximum depth [m]" -> [_ w416]
                  tunnel: w385 -> [w396 _]
                  frame #0 {
                    n152 = case shown="True" w396 {
                      frame #0 {
                      }
                      frame #1 {
                        n153 = property on="isMaxPaySet" class="Bool (strict)"() -> ("Value"=w402:bool)  [unwired: 2 in, 2 out]
                        n154 = Not(x=w402) -> (.not. x?=w401:bool)
                        n155 = property on="Payout" class="Slide (strict)"() -> ("Value"=w404:dbl)  [unwired: 2 in, 2 out]
                        n156 = property on="Maximum payout [turns]" class="DigNum (strict)"() -> ("Value"=w403:dbl)  [unwired: 2 in, 2 out]
                        n157 = property on="Velocity Now" class="Knob (strict)"() -> ("Value"=w400:dbl)  [unwired: 2 in, 2 out]
                        n158 = Less?(x=w404, y=w403) -> (x < y?=w397:bool)
                        n159 = Greater Or Equal To 0?(x=w400) -> (x >= 0?=w398:bool)
                        n160 = And(x=w398, y=w397) -> (x .and. y?=w399:bool)
                        n161 = case shown="True" w401 {
                          selector: w401 -> [_ w405]
                          frame #0 {
                          }
                          frame #1 {
                            n162 = property on="isMaxPaySet" class="Bool (strict)"("Val(Sgnl)"=w405) -> ()  [unwired: 2 in, 2 out]
                            n163 = property on="Maximum payout [turns]" class="DigNum (strict)"() -> ("Value"=→"Old Max Payout":dbl)  [unwired: 2 in, 2 out]
                          }
                        }
                        n164 = case shown="True" w399 {
                          tunnel: w404 -> [_ w408]
                          frame #0 {
                          }
                          frame #1 {
                            n165 = Multiply(x=w408, y=0.8) -> (x*y=w407:dbl)
                            n166 = property on="Maximum payout [turns]" class="DigNum (strict)"("Val(Sgnl)"=w407) -> ()  [unwired: 2 in, 2 out]
                          }
                        }
                      }
                    }
                  }
                  frame #1 {
                    n167 = property on="Velocity Now" class="Knob (strict)"() -> ("Value"=w419:dbl)  [unwired: 2 in, 2 out]
                    n168 = property on="isMaxPaySet" class="Bool (strict)"() -> ("Value"=w412:bool)  [unwired: 2 in, 2 out]
                    n169 = Multiply(x=w416, y=0.8) -> (x*y=w415:dbl)
                    n170 = Greater?(x=w414, y=w415) -> (0:w413:bool)
                    n171 = Less Than 0?(x=w419) -> (x < 0?=w418:bool)
                    n172 = And(x=w418, y=w413) -> (x .and. y?=w411:bool)
                    n173 = And(x=w412, y=w411) -> (x .and. y?=w410:bool)
                    n174 = case shown="True" w410 {
                      selector: w410 -> [_ w421]
                      frame #0 {
                      }
                      frame #1 {
                        n175 = Not(x=w421) -> (.not. x?=w420:bool)
                        n176 = property on="isMaxPaySet" class="Bool (strict)"("Val(Sgnl)"=w420) -> ()  [unwired: 2 in, 2 out]
                        n177 = property on="Old Max Payout" class="DigNum (strict)"() -> ("Value"=w422:dbl)  [unwired: 2 in, 2 out]
                        n178 = property on="Maximum payout [turns]" class="DigNum (strict)"("Val(Sgnl)"=w422) -> ()  [unwired: 2 in, 2 out]
                      }
                    }
                  }
                }
                n179 = Less?(x=w379, y=w374) -> (x < y?=w378:bool)
                n180 = And(x=w376, y=w378) -> (x .and. y?=w377:bool)
                n181 = case shown="False" w376 {
                  frame #0 {
                    n182 = property on="Max depth" class="DigNum (strict)"("Value"=0.0) -> ()  [unwired: 2 in, 2 out]
                  }
                  frame #1 {
                  }
                }
                n183 = case shown="True" w377 {
                  tunnel: w374 -> [_ w425]
                  frame #0 {
                  }
                  frame #1 {
                    n184 = Get Date/Time In Seconds() -> (seconds since 1Jan1904=→"Time @ max":timestamp)
                    n185 = property on="Payout" class="Slide (strict)"() -> ("Value"=→"Max payout":dbl)  [unwired: 2 in, 2 out]
                    "Max depth" <- w425
                  }
                }
              }
              frame #1 {
                # "If CTD is emtpy string: increment CTD Miss count, and blink CTD bar"
                n186 = property on="CTD Com Miss Count" class="DigNum (strict)"() -> ("Value"=w430:dbl)  [unwired: 2 in, 2 out]
                n187 = Increment(x=w430) -> (x+1=w428:dbl)
                n188 = Greater?(x=w428, y=1) -> (0:w426:bool)
                n189 = property on="CTD data" class="String"("Blinking"=w426) -> ()  [unwired: 2 in, 2 out]
                n190 = property on="Depth" class="Slide (strict)"("Blinking"=w426) -> ()  [unwired: 2 in, 2 out]
                n191 = property on="CTD Com Miss Count" class="DigNum (strict)"("Value"=w428) -> ()  [unwired: 2 in, 2 out]
                n192 = property on="Pressure" class="WFChart (strict)"("Blinking"=w426) -> ()  [unwired: 2 in, 2 out]
                n193 = property on="Depth Derivative" class="WFChart (strict)"("Blinking"=w426) -> ()  [unwired: 2 in, 2 out]
                n194 = property on="Conductivity" class="WFChart (strict)"("Blinking"=w426) -> ()  [unwired: 2 in, 2 out]
                n195 = property on="Temperature" class="WFChart (strict)"("Blinking"=w426) -> ()  [unwired: 2 in, 2 out]
              }
            }
            n196 = Bundle("Depth in meters"=w366, "Value"=w372) -> (→"Depth History":cluster{"Depth in meters":dbl, "Value":dbl})  [unwired: 1 in]
          }
        }
      }
      frame #7 {
        # "Check for dead com links"
        n197 = stacked-sequence {
          seq-local: [w438 _] -> [_ w455]
          tunnel: w436 -> [w439 _]
          tunnel: [_ w455] -> w435
          tunnel: w434 -> [_ w456]
          tunnel: [_ w454] -> w433
          tunnel: w432 -> [w437 _]
          frame #0 {
            # "If winch miss count > 25, close connection and open again"
            n198 = property on="Winch Com Miss Count" class="DigNum (strict)"() -> ("Value"=w442:dbl)  [unwired: 2 in, 2 out]
            n199 = Greater?(x=w442, y=25) -> (0:w440:bool)
            n200 = case shown="True" w440 {
              tunnel: w439 -> [w443 w446]
              tunnel: [w443 w445] -> w438
              tunnel: w437 -> [_ w444]
              frame #0 {
              }
              frame #1 {
                n201 = stacked-sequence {
                  tunnel: w446 -> [w448 _ _]
                  tunnel: [_ _ w451] -> w445
                  tunnel: w444 -> [_ _ w449]
                  frame #0 {
                    n202 = TCP Close Connection(connection ID=w448) -> (error out=w447:errorcluster)  [unwired: 2 in, 1 out]
                    n203 = call <vilib>:"Clear Errors.vi"("error in (no error)"=w447) -> ()  [unwired: 6 in, 1 out]
                  }
                  frame #1 {
                    n204 = call "Time Delay"() -> ()  [unwired: 11 in, 1 out]
                  }
                  frame #2 {
                    n205 = TCP Open Connection(address=w449, remote port or service name=4050, timeout ms (60000)=1000) -> (connection ID=w451:refnum<k5>, error out=w450:errorcluster)  [unwired: 2 in]
                    n206 = call <vilib>:"Clear Errors.vi"("error in (no error)"=w450) -> ()  [unwired: 6 in, 1 out]
                  }
                }
              }
            }
          }
          frame #1 {
            # "If CTD miss count > 10, close connection and open again"
            n207 = property on="CTD Com Miss Count" class="DigNum (strict)"() -> ("Value"=w457:dbl)  [unwired: 2 in, 2 out]
            n208 = Greater?(x=w457, y=10) -> (0:w459:bool)
            n209 = case shown="True" w459 {
              tunnel: w456 -> [w460 w462]
              tunnel: [w460 w461] -> w454
              frame #0 {
              }
              frame #1 {
                n210 = stacked-sequence {
                  tunnel: w462 -> [w464 _ _ _]
                  tunnel: [_ _ _ w469] -> w461
                  frame #0 {
                    n211 = TCP Close Connection(connection ID=w464) -> (error out=w463:errorcluster)  [unwired: 2 in, 1 out]
                    n212 = call <vilib>:"Clear Errors.vi"("error in (no error)"=w463) -> ()  [unwired: 6 in, 1 out]
                  }
                  frame #1 {
                    n213 = call "Time Delay2"() -> ()  [unwired: 11 in, 1 out]
                  }
                  frame #2 {
                    n214 = property on="CTD Com Miss Count" class="DigNum (strict)"("Value"=0) -> ()  [unwired: 2 in, 2 out]
                  }
                  frame #3 {
                    n215 = property on="Port" class="DigNum (strict)"() -> ("Value"=w467:i32)  [unwired: 2 in, 2 out]
                    n216 = property on="CTD Data  IP Address" class="Str"() -> ("Value"=w468:string)  [unwired: 2 in, 2 out]
                    n217 = TCP Open Connection(address=w468, remote port or service name=w467, timeout ms (60000)=1000) -> (connection ID=w469:refnum<k5>, error out=w466:errorcluster)  [unwired: 2 in]
                    n218 = call <vilib>:"Clear Errors.vi"("error in (no error)"=w466) -> ()  [unwired: 6 in, 1 out]
                  }
                }
              }
            }
          }
        }
      }
      frame #8 {
        # "Check if the values set by the user \nand the values on the controls are the same"
        # "Image Capture of the Front Panel"
        n219 = property on="Enabled" class="Bool (strict)"() -> ("Value"=w471:bool)  [unwired: 2 in, 2 out]
        n220 = case shown="True" w471 {
          frame #0 {
          }
          frame #1 {
            n221 = property on="Min Payout" class="DigNum (strict)"() -> ("Value"=w510:dbl)  [unwired: 2 in, 2 out]
            n222 = property on="Minimum payout [turns]" class="DigNum (strict)"() -> ("Value"=w509:dbl)  [unwired: 2 in, 2 out]
            n223 = property on="Wire In Speed" class="DigNum (strict)"() -> ("Value"=w502:dbl)  [unwired: 2 in, 2 out]
            n224 = property on="Wire In Speed\n[turns/sec]" class="DigNum (strict)"() -> ("Value"=w501:dbl)  [unwired: 2 in, 2 out]
            n225 = property on="Maximum payout [turns]" class="DigNum (strict)"() -> ("Value"=w508:dbl)  [unwired: 2 in, 2 out]
            n226 = property on="Max Payout" class="DigNum (strict)"() -> ("Value"=w507:dbl)  [unwired: 2 in, 2 out]
            n227 = property on="Wire Out Speed\n[turns/sec]" class="DigNum (strict)"() -> ("Value"=w505:dbl)  [unwired: 2 in, 2 out]
            n228 = property on="Wire Out Speed" class="DigNum (strict)"() -> ("Value"=w504:dbl)  [unwired: 2 in, 2 out]
            n229 = Not Equal?(x=w509, y=w510) -> (x != y?=w511:bool)
            n230 = Not Equal?(x=w502, y=w501) -> (x != y?=w500:bool)
            n231 = Not Equal?(x=w508, y=w507) -> (x != y?=w506:bool)
            n232 = Not Equal?(x=w505, y=w504) -> (x != y?=w503:bool)
            n233 = property on="Minimum payout [turns]" class="DigNum (strict)"("Blinking"=w511) -> ()  [unwired: 2 in, 2 out]
            n234 = property on="Min Payout" class="DigNum (strict)"("Blinking"=w511) -> ()  [unwired: 2 in, 2 out]
            n235 = property on="Wire In Speed\n[turns/sec]" class="DigNum (strict)"("Blinking"=w500) -> ()  [unwired: 2 in, 2 out]
            n236 = property on="Maximum payout [turns]" class="DigNum (strict)"("Blinking"=w506) -> ()  [unwired: 2 in, 2 out]
            n237 = property on="Wire Out Speed\n[turns/sec]" class="DigNum (strict)"("Blinking"=w503) -> ()  [unwired: 2 in, 2 out]
            n238 = property on="Wire In Speed" class="DigNum (strict)"("Blinking"=w500) -> ()  [unwired: 2 in, 2 out]
            n239 = property on="Max Payout" class="DigNum (strict)"("Blinking"=w506) -> ()  [unwired: 2 in, 2 out]
            n240 = property on="Wire Out Speed" class="DigNum (strict)"("Blinking"=w503) -> ()  [unwired: 2 in, 2 out]
            n241 = property on="Stop decel out" class="DigNum (strict)"() -> ("Value"=w478:dbl)  [unwired: 2 in, 2 out]
            n242 = property on="Decel Stop Out" class="DigNum (strict)"() -> ("Value"=w477:dbl)  [unwired: 2 in, 2 out]
            n243 = property on="Final in Speed" class="DigNum (strict)"() -> ("Value"=w499:dbl)  [unwired: 2 in, 2 out]
            n244 = property on="Final In Speed\n[turns/sec]" class="DigNum (strict)"() -> ("Value"=w498:dbl)  [unwired: 2 in, 2 out]
            n245 = property on="Acc Out" class="DigNum (strict)"() -> ("Value"=w490:dbl)  [unwired: 2 in, 2 out]
            n246 = property on="Accel out" class="DigNum (strict)"() -> ("Value"=w489:dbl)  [unwired: 2 in, 2 out]
            n247 = property on="Acc In" class="DigNum (strict)"() -> ("Value"=w493:dbl)  [unwired: 2 in, 2 out]
            n248 = property on="Accel  in" class="DigNum (strict)"() -> ("Value"=w492:dbl)  [unwired: 2 in, 2 out]
            n249 = Not Equal?(x=w478, y=w477) -> (x != y?=w476:bool)
            n250 = Not Equal?(x=w499, y=w498) -> (x != y?=w497:bool)
            n251 = Not Equal?(x=w490, y=w489) -> (x != y?=w488:bool)
            n252 = Not Equal?(x=w493, y=w492) -> (x != y?=w491:bool)
            n253 = property on="Stop decel out" class="DigNum (strict)"("Blinking"=w476) -> ()  [unwired: 2 in, 2 out]
            n254 = property on="Decel Stop Out" class="DigNum (strict)"("Blinking"=w476) -> ()  [unwired: 2 in, 2 out]
            n255 = property on="Final in Speed" class="DigNum (strict)"("Blinking"=w497) -> ()  [unwired: 2 in, 2 out]
            n256 = property on="Final In Speed\n[turns/sec]" class="DigNum (strict)"("Blinking"=w497) -> ()  [unwired: 2 in, 2 out]
            n257 = property on="Accel out" class="DigNum (strict)"("Blinking"=w488) -> ()  [unwired: 2 in, 2 out]
            n258 = property on="Accel  in" class="DigNum (strict)"("Blinking"=w491) -> ()  [unwired: 2 in, 2 out]
            n259 = property on="Acc Out" class="DigNum (strict)"("Blinking"=w488) -> ()  [unwired: 2 in, 2 out]
            n260 = property on="Acc In" class="DigNum (strict)"("Blinking"=w491) -> ()  [unwired: 2 in, 2 out]
            n261 = property on="Decel Stop In" class="DigNum (strict)"() -> ("Value"=w481:dbl)  [unwired: 2 in, 2 out]
            n262 = property on="Stop decel in" class="DigNum (strict)"() -> ("Value"=w480:dbl)  [unwired: 2 in, 2 out]
            n263 = property on="Decel in" class="DigNum (strict)"() -> ("Value"=w487:dbl)  [unwired: 2 in, 2 out]
            n264 = property on="Decel In" class="DigNum (strict)"() -> ("Value"=w486:dbl)  [unwired: 2 in, 2 out]
            n265 = property on="Decel Out" class="DigNum (strict)"() -> ("Value"=w484:dbl)  [unwired: 2 in, 2 out]
            n266 = property on="Decel out" class="DigNum (strict)"() -> ("Value"=w483:dbl)  [unwired: 2 in, 2 out]
            n267 = property on="Slow Depth" class="DigNum (strict)"() -> ("Value"=w496:dbl)  [unwired: 2 in, 2 out]
            n268 = property on="Slow depth\n[turns]" class="DigNum (strict)"() -> ("Value"=w495:dbl)  [unwired: 2 in, 2 out]
            n269 = Not Equal?(x=w481, y=w480) -> (x != y?=w479:bool)
            n270 = Not Equal?(x=w487, y=w486) -> (x != y?=w485:bool)
            n271 = Not Equal?(x=w484, y=w483) -> (x != y?=w482:bool)
            n272 = Not Equal?(x=w496, y=w495) -> (x != y?=w494:bool)
            n273 = property on="Stop decel in" class="DigNum (strict)"("Blinking"=w479) -> ()  [unwired: 2 in, 2 out]
            n274 = property on="Decel in" class="DigNum (strict)"("Blinking"=w485) -> ()  [unwired: 2 in, 2 out]
            n275 = property on="Decel out" class="DigNum (strict)"("Blinking"=w482) -> ()  [unwired: 2 in, 2 out]
            n276 = property on="Decel Stop In" class="DigNum (strict)"("Blinking"=w479) -> ()  [unwired: 2 in, 2 out]
            n277 = property on="Decel In" class="DigNum (strict)"("Blinking"=w485) -> ()  [unwired: 2 in, 2 out]
            n278 = property on="Decel Out" class="DigNum (strict)"("Blinking"=w482) -> ()  [unwired: 2 in, 2 out]
            n279 = property on="Slow depth\n[turns]" class="DigNum (strict)"("Blinking"=w494) -> ()  [unwired: 2 in, 2 out]
            n280 = property on="Slow Depth" class="DigNum (strict)"("Blinking"=w494) -> ()  [unwired: 2 in, 2 out]
          }
        }
        n281 = Get Date/Time In Seconds() -> (seconds since 1Jan1904=w475:timestamp)
        n282 = Format Date/Time String(seconds (now)=w475) -> (date/time string=w474:string)  [unwired: 2 in]
        n283 = Concatenate Strings("Updated: ", w474) -> (→"Last update string":string)
      }
    }
  }
  n284 = TCP Close Connection(connection ID=w9, error in (no error)=w42) -> (error out=w11:errorcluster)  [unwired: 1 in, 1 out]
  n285 = TCP Close Connection(connection ID=w18, error in (no error)=w16) -> (error out=w20:errorcluster)  [unwired: 1 in, 1 out]
  n286 = call <vilib>:"Simple Error Handler.vi"("error in (no error)"=w11) -> ()  [unwired: 4 in, 5 out]
  n287 = call <vilib>:"Simple Error Handler.vi"("error in (no error)"=w20) -> ()  [unwired: 4 in, 5 out]
  "CTD Com Miss Count" <- w10
  "Winch Com Miss Count" <- w10
  "isMaxPaySet" <- FALSE
  "RL Status Received" <- FALSE
